vi "Day 12-Create Map.vi"(11 "Connections in":string[][](array[string])) -> (3 "Map":map{string, set{string}}(c390))   [LabVIEW 2021]
uses:
  <vilib>/Utility/miscctls.llb/LVMapReplaceAction.ctl
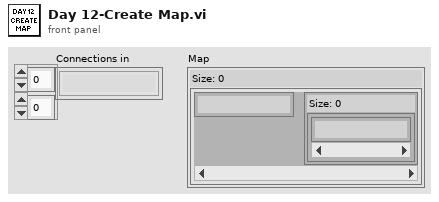
[diagram p1: front panel]
types:
  T1 = typedef "LVMapReplaceAction.ctl" = enum32{"Modify Entry only if found", "Add or Modify Entry", "Delete Entry"}
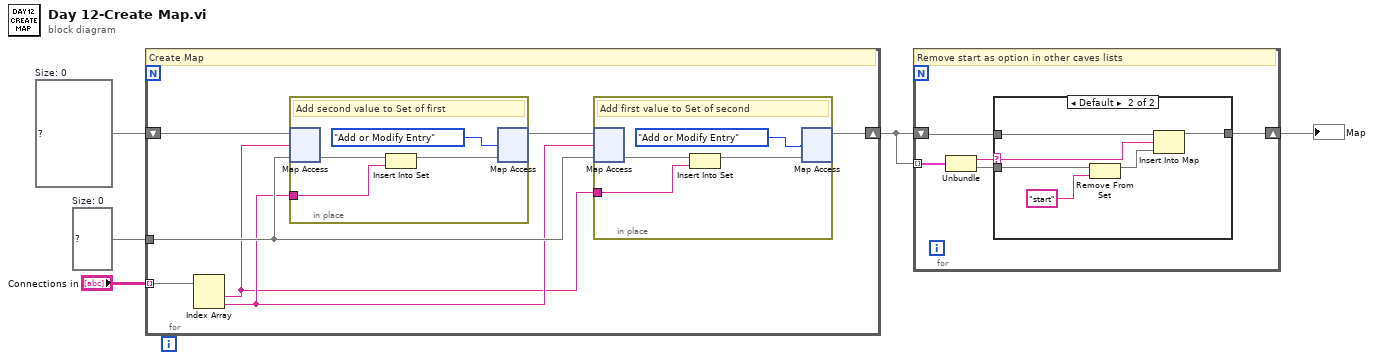
[diagram p0: block diagram]
diagram:
  w5 = set{string} {}  # Size: 0
  w4 = map{string, set{string}} {}  # Size: 0
  n1 = for {
    tunnel: "Connections in" -> [w12] mode=indexing
    shift-right: [w8] -> w2
    shift-left: w4 -> [w11]
    tunnel: w5 -> [w9]
    # "Create Map"
    n2 = Index Array(array=w12) -> (element #1=w6:string, element #2=w7:string)  [unwired: 2 in]
    n3 = in-place {
      in-place-border: w7 -> [w19]
      # "Add second value to Set of first"
      n4 = in-place-map #1(w11, w6, w9) -> (w20:set{string})  [unwired: 1 out]
      n5 = Insert Into Set(10:w19, 11:w20) -> (3:w18:set{string})  [unwired: 1 out]
      n6 = in-place-map #1(w18, LVMapReplaceAction."Add or Modify Entry" ("action")) -> (w10:map{string, set{string}})  [unwired: 2 out]
    }
    n7 = in-place {
      in-place-border: w6 -> [w14]
      # "Add first value to Set of second"
      n8 = in-place-map #2(w10, w7, w9) -> (w16:set{string})  [unwired: 1 out]
      n9 = Insert Into Set(10:w14, 11:w16) -> (3:w15:set{string})  [unwired: 1 out]
      n10 = in-place-map #2(w15, LVMapReplaceAction."Add or Modify Entry" ("action")) -> (w8:map{string, set{string}})  [unwired: 2 out]
    }
  }
  n11 = for {
    tunnel: w2 -> [w25] mode=indexing
    shift-right: [w22] -> w1
    shift-left: w2 -> [w23]
    # "Remove start as option in other caves lists"
    n12 = Unbundle(w25) -> ("String"=w24:string, w21:set{string})
    n13 = case shown="Default" w24 {
      selector: w24 -> [_ w27]
      tunnel: w23 -> [w26 w32]
      tunnel: [w26 w31] -> w22
      tunnel: w21 -> [_ w30]
      frame "start" {
      }
      frame Default {
        n14 = Remove From Set(10:"start", 11:w30) -> (3:w28:set{string})  [unwired: 1 out]
        n15 = Insert Into Map(map in=w32, key=w27, value=w28) -> (map out=w31:map{string, set{string}})  [unwired: 2 out]
      }
    }
  }
  "Map" <- w1
